vi "CMD_GOTOIFN.vi"(6 "Gantry in":refnum<class "Gantry.lvclass">, 8 "error in (no error)":errorcluster, 10 "Arguments":string[](array[string]), 11 "gScript Interpreter in":refnum<class "gScript Interpreter.lvclass">) -> (0 "error out":errorcluster, 3 "gScript Interpreter out":refnum<class "gScript Interpreter.lvclass">, 4 "Gantry out":refnum<class "Gantry.lvclass">)   [LabVIEW 2022 SP3, in "gScript Interpreter.lvclass"]
uses:
  gScript Interpreter.lvclass
  gScript Interpreter.lvclass/gScript Interpreter.ctl
  Shared Components/Gantry Class/Gantry.lvclass
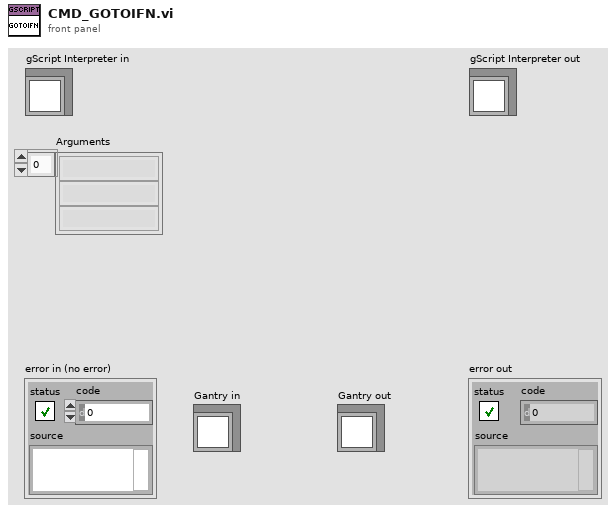
[diagram p1: front panel]
types:
  T1 = typedef "Memory Cell.ctl" = cluster{"type":T2, "x":dbl, "y":dbl, "z":dbl, "w":dbl}
  T2 = typedef "Memory Cell Type Enum.ctl" = enum16{"integer", "float", "vector", "rotation"}
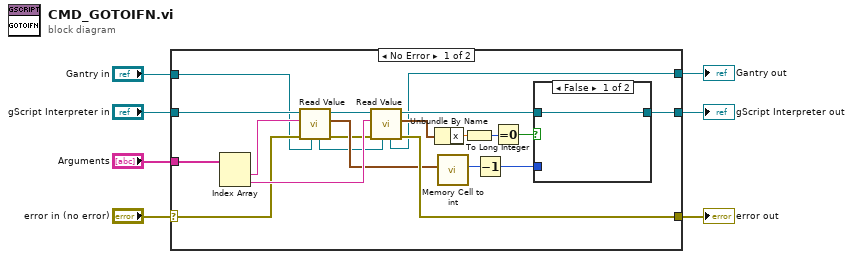
[diagram p0: block diagram]
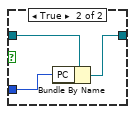
[diagram p2: hidden frame]
diagram:
  n1 = case shown="No Error" "error in (no error)" {
    selector: "error in (no error)" -> [w14 w34]
    tunnel: [w20 w34] -> w6
    tunnel: [w18 w33] -> w4
    tunnel: "gScript Interpreter in" -> [w16 w33]
    tunnel: "Arguments" -> [w27 _]
    tunnel: "Gantry in" -> [w10 w32]
    tunnel: [w8 w32] -> w1
    frame No Error {
      n2 = Index Array(array=w27) -> (element #1=w12:string, element #2=w25:string)  [unwired: 2 in]
      n3 = call-dynamic "Read Value.vi"("Gantry in"=w10, "error in (no error)"=w14, "String in"=w12, "gScript Interpreter in"=w16) -> ("error out"=w13:errorcluster, "Memory Cell"=w17:T1, "gScript Interpreter out"=w15:refnum<class "gScript Interpreter.lvclass">, "Gantry out"=w9:refnum<class "Gantry.lvclass">)  [unwired: 4 in]
      n4 = call-dynamic "Read Value.vi"("Gantry in"=w9, "error in (no error)"=w13, "String in"=w25, "gScript Interpreter in"=w15) -> ("error out"=w20:errorcluster, "Memory Cell"=w24:T1, "gScript Interpreter out"=w19:refnum<class "gScript Interpreter.lvclass">, "Gantry out"=w8:refnum<class "Gantry.lvclass">)  [unwired: 4 in]
      n5 = Unbundle By Name(w24) -> ("x"=w23:dbl)
      n6 = call "Memory Cell to int.vi"("Memory Cell"=w17) -> ("Int out"=w11:i32)  [unwired: 10 in]
      n7 = To Long Integer(number=w23) -> (32bit integer=w22:i32)
      n8 = Decrement(x=w11) -> (x-1=w26:i32)
      n9 = Equal To 0?(x=w22) -> (x = 0?=w21:bool)
      n10 = case shown="False" w21 {
        tunnel: w26 -> [_ w31]
        tunnel: w19 -> [w28 w30]
        tunnel: [w28 w29] -> w18
        frame False {
        }
        frame True {
          n11 = Bundle By Name(cluster=w30, "PC"=w31) -> (w29:refnum<class "gScript Interpreter.lvclass">)
        }
      }
    }
    frame Error {
    }
  }
  "error out" <- w6
  "gScript Interpreter out" <- w4
  "Gantry out" <- w1
